vi "H5LTmake_dataset.vi"(2 "Array":variant, 3 "loc_id":i32, 7 "name":string, 9 "error in (no error)":errorcluster) -> (6 "error out":errorcluster)   [LabVIEW 2009]
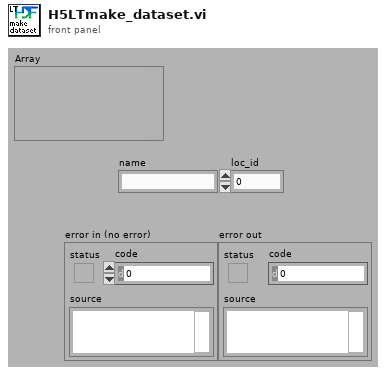
[diagram p1: front panel]
types:
  T1 = typedef "Type Descriptor Enumeration__ogtk.ctl" = enum8{"<Null>", "I8", "I16", "I32", "I64", "U8", "U16", "U32", "U64", "SGL", "DBL", "EXT", "CSG", "CDB", "CXT", "0x0F", "0x10", "0x11", "0x12", "0x13", "0x14", "Enum U8", "Enum U16", "Enum U32", "Enum U64", "SGL PQ", "DBL PQ", "EXT PQ", "CSG PQ", "CDB PQ", "CXT PQ", "0x1F", "0x20", "Boolean", "0x22", "0x23", "0x24", "0x25", "0x26", "0x27", "0x28", "0x29", "0x2A", "0x2B", "0x2C", "0x2D", "0x2E", "0x2F", "String", "0x31", "Path", "Pict", "0x34", "0x35", "0x36", "DAQ", "0x38", "0x39", "0x3A", "0x3B", "0x3C", "0x3D", "0x3E", "0x3F", "Array", "0x41", "0x42", "0x43", "0x44", "0x45", "0x46", "0x47", "0x48", "0x49", "0x4A", "0x4B", "0x4C", "0x4D", "0x4E", "0x4F", "Cluster", "0x51", "0x52", "Variant", "Waveform", "0x55", "0x56", "0x57", "0x58", "0x59", "0x5A", "0x5B", "0x5C", "0x5D", "0x5E", "0x5F", "0x60", "0x61", "0x62", "0x63", "0x64", "0x65", "0x66", "0x67", "0x68", "0x69", "0x6A", "0x6B", "0x6C", "0x6D", "0x6E", "0x6F", "Refnum"}
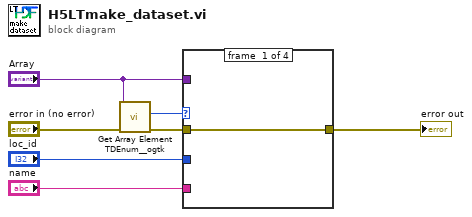
[diagram p0: block diagram]
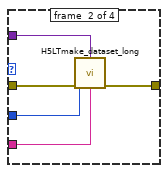
[diagram p2: hidden frame]
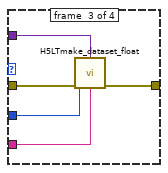
[diagram p3: hidden frame]
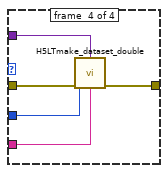
[diagram p4: hidden frame]
diagram:
  n1 = call <userlib>:"Get Array Element TDEnum__ogtk.vi"("error in (no error)"="error in (no error)", "Array"="Array") -> ("error out"=w6:errorcluster, "Element Type"=w5:T1)  [unwired: 8 in]
  n2 = case shown="\"DBL\"" w5 {
    tunnel: w6 -> [w8 w13 w18 w23]
    tunnel: "name" -> [_ w12 w16 w21]
    tunnel: "loc_id" -> [_ w11 w14 w19]
    tunnel: "Array" -> [_ w10 w15 w20]
    tunnel: [w8 w9 w17 w22] -> w1
    frame #0 {
    }
    frame #1 {
      n3 = call "H5LTmake_dataset_long.vi"("I32 Array"=w10, "loc_id"=w11, "name"=w12, "error in (no error)"=w13) -> ("error out"=w9:errorcluster)  [unwired: 5 in]
    }
    frame #2 {
      n4 = call "H5LTmake_dataset_float.vi"("SGL Array"=w15, "loc_id"=w14, "name"=w16, "error in (no error)"=w18) -> ("error out"=w17:errorcluster)  [unwired: 5 in]
    }
    frame #3 {
      n5 = call "H5LTmake_dataset_double.vi"("DBL Array"=w20, "loc_id"=w19, "name"=w21, "error in (no error)"=w23) -> ("error out"=w22:errorcluster)  [unwired: 5 in]
    }
  }
  "error out" <- w1
